vi "ke37xx Configure Digital I-O.vi"(0 "VISA Resource Name":refnum<visa-resource-name>, 5 "Line (1)":u8=1 min=1 max=14, 7 "Stimulus (0: None)":T2(ring), 9 "Pulse Width (10 sec)":dbl=10.0, 11 "error in (no error)":errorcluster, 12 "Mode (0: Falling Edge)":T1(ring)) -> (4 "VISA Resource Name Out":refnum<visa-resource-name>, 15 "error out":errorcluster)   [LabVIEW 2009, in "Keithley 3700 Series.lvlib"]
doc: "This VI allows you to configure various aspects of a specific digital I/O line. You can control the pulse width and the mode in which the line operations. You can also set the stimulus that causes the line to enter the detected state."
uses:
  <instrlib>/Keithley 3706/Keithley 3700 Series.lvlib
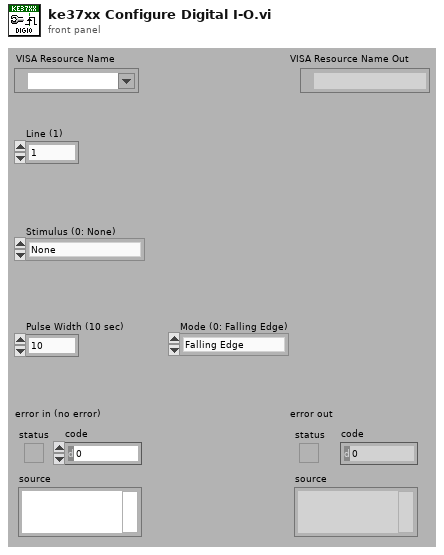
[diagram p1: front panel]
types:
  T1 = enum16{"Falling Edge", "Rising Edge", "Falling or Rising Edge", "Synchronous"}
  T2 = enum16{"None", "Alarm 1", "Alarm 2", "Digital I/O Line 1", "Digital I/O Line 2", "Digital I/O Line 3", "Digital I/O Line 4", "Digital I/O Line 5", "Digital I/O Line 6", "Digital I/O Line 7", "Digital I/O Line 8", "Digital I/O Line 9", "Digital I/O Line 10", "Digital I/O Line 11", "Digital I/O Line 12", "Digital I/O Line 13", "Digital I/O Line 14", "TSP Link Line 1", "TSP Link Line 2", "TSP Link Line 3", "Blender 1", "Blender 2", "Timer 1", "Timer 2", "Timer 3", "Timer 4", "LAN Line 1", "LAN Line 2", "LAN Line 3", "LAN Line 4", "LAN Line 5", "LAN Line 6", "LAN Line 7", "LAN Line 8", "DMM Limit 1 High", "DMM Limit 1 Low", "DMM Limit 2 High", "DMM Limit 2 Low", "Display", "Measure Complete", "Sequence Complete", "Scan Ready", "Scan Start", "Scan Complete", "Channel Ready", "Idle", "Software"}
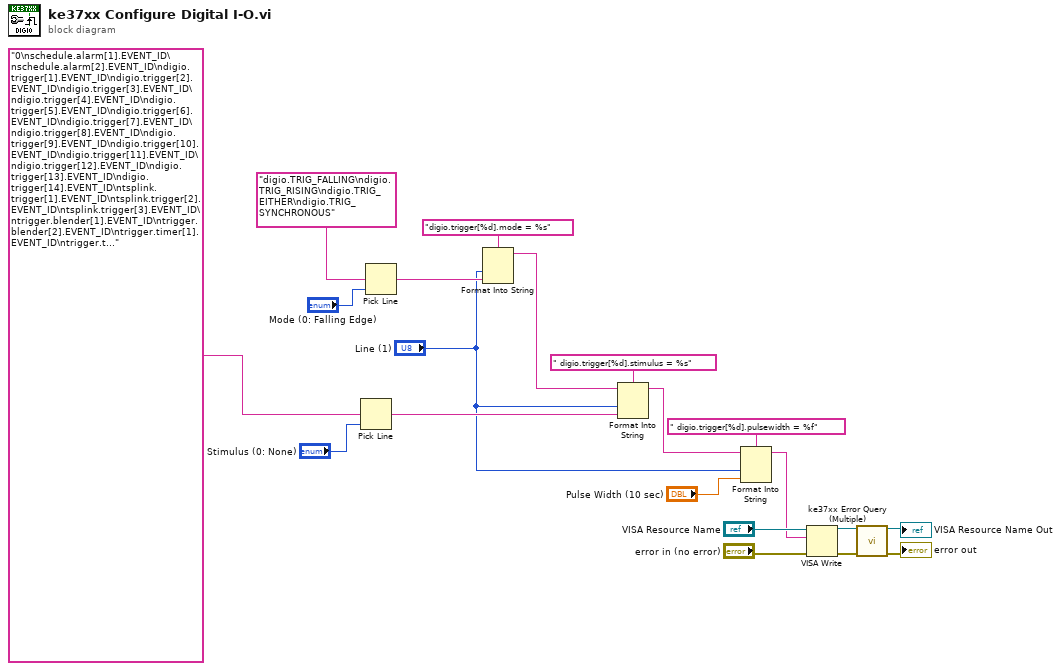
[diagram p0: block diagram]
diagram:
  n1 = Pick Line(multi-line string="0\nschedule.alarm[1].EVENT_ID\nschedule.alarm[2].EVENT_ID\ndigio.trigger[1].EVENT_ID\ndigio.trigger[2].EVENT_ID\ndigio.trigger[3].EVENT_ID\ndigio.trigger[4].EVENT_ID\ndigio.trigger[5].EVENT_ID\ndigio.trigger[6].EVENT_ID\ndigio.trigger[7].EVENT_ID\ndigio.trigger[8].EVENT_ID\ndigio.trigger[9].EVENT_ID\ndigio.trigger[10].EVENT_ID\ndigio.trigger[11].EVENT_ID\ndigio.trigger[12].EVENT_ID\ndigio.trigger[13].EVENT_ID\ndigio.trigger[14].EVENT_ID\ntsplink.trigger[1].EVENT_ID\ntsplink.trigger[2].EVENT_ID\ntsplink.trigger[3].EVENT_ID\ntrigger.blender[1].EVENT_ID\ntrigger.blender[2].EVENT_ID\ntrigger.timer[1].EVENT_ID\ntrigger.timer[2].EVENT_ID\ntrigger.timer[3].EVENT_ID\ntrigger.timer[4].EVENT_ID\nlan.trigger[1].EVENT_ID\nlan.trigger[2].EVENT_ID\nlan.trigger[3].EVENT_ID\nlan.trigger[4].EVENT_ID\nlan.trigger[5].EVENT_ID\nlan.trigger[6].EVENT_ID\nlan.trigger[7].EVENT_ID\nlan.trigger[8].EVENT_ID\ndmm.trigger.EVENT_LIMIT1_HIGH\ndmm.trigger.EVENT_LIMIT1_LOW\ndmm.trigger.EVENT_LIMIT2_HIGH\ndmm.trigger.EVENT_LIMIT2_LOW\ndisplay.trigger.EVENT_ID\nscan.trigger.EVENT_MEASURE_COMP\nscan.trigger.EVENT_SEQUENCE_COMP\nscan.trigger.EVENT_SCAN_READY\nscan.trigger.EVENT_SCAN_START\nscan.trigger.EVENT_SCAN_COMP\nscan.trigger.EVENT_CHANNEL_READY\nscan.trigger.EVENT_IDLE\ntrigger.EVENT_ID", line index="Stimulus (0: None)") -> (output string=w6:string)  [unwired: 1 out]
  n2 = Pick Line(multi-line string="digio.TRIG_FALLING\ndigio.TRIG_RISING\ndigio.TRIG_EITHER\ndigio.TRIG_SYNCHRONOUS", line index="Mode (0: Falling Edge)") -> (output string=w9:string)  [unwired: 1 out]
  n3 = Format Into String(format string="digio.trigger[%d].mode = %s", "Line (1)", w9) -> (resulting string=w4:string)  [unwired: 2 in, 1 out]
  n4 = Format Into String(format string=" digio.trigger[%d].stimulus = %s", initial string=w4, "Line (1)", w6) -> (resulting string=w5:string)  [unwired: 1 in, 1 out]
  n5 = Format Into String(format string=" digio.trigger[%d].pulsewidth = %f", initial string=w5, "Line (1)", "Pulse Width (10 sec)") -> (resulting string=w1:string)  [unwired: 1 in, 1 out]
  n6 = VISA Write(VISA resource name="VISA Resource Name", write buffer=w1, error in (no error)="error in (no error)") -> (VISA resource name out=w16:refnum<visa-resource-name>, error out=w15:errorcluster)  [unwired: 1 out]
  n7 = call <instrlib>:"ke37xx Error Query (Multiple).vi"("VISA resource name"=w16, "error in (no error)"=w15) -> ("VISA resource name out"=→"VISA Resource Name Out":refnum<visa-resource-name>, "error out"=→"error out":errorcluster)  [unwired: 12 out]
